vi "Day 13.vi"() -> ()   [LabVIEW 2021]
panel:
  out "output 2":bool[][](array[boolean])
  out "input":string
  out "input file":path
  in  "Run [T]/ Example[F]":bool
  out "ouptut 1":u32
  # "Advent of Code 2021 - Day 11 - Dumbo Octopus"
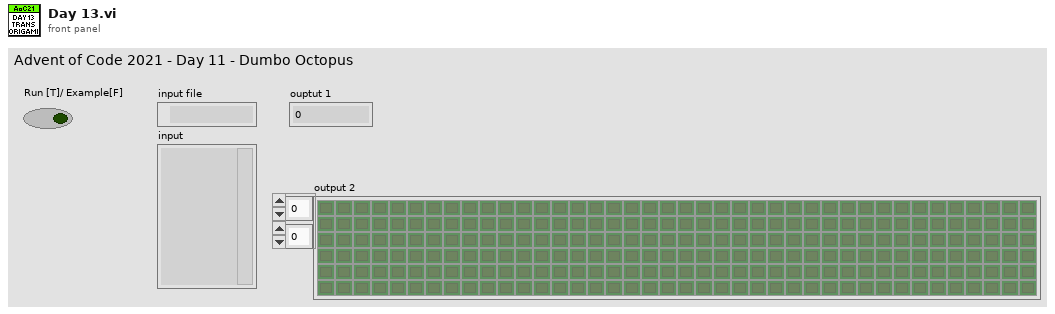
[diagram p1: front panel]
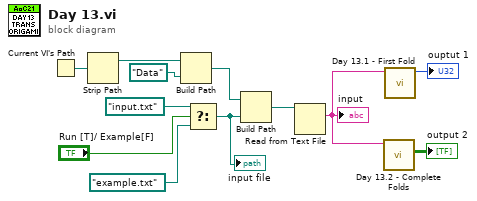
[diagram p0: block diagram]
diagram:
  n1 = Current VI's Path() -> (path=w12:path)
  n2 = Strip Path(path=w12) -> (stripped path=w11:path)  [unwired: 1 out]
  n3 = Build Path(base path=w11, name or relative path=path "Data") -> (appended path=w9:path)
  n4 = Select(t=path "input.txt" ("name or relative path"), s="Run [T]/ Example[F]", f=path "example.txt" ("name or relative path")) -> (s? t:f=w5:path)
  "input file" <- w5
  n5 = Build Path(base path=w9, name or relative path=w5) -> (appended path=w3:path)
  n6 = Read from Text File(file (use dialog)=w3) -> (text=w2:string)  [unwired: 3 in, 3 out]
  "input" <- w2
  n7 = call "Day 13.2 - Complete Folds.vi"("input"=w2) -> ("output array"=→"output 2":bool[][])  [unwired: 9 in, 1 out]
  n8 = call "Day 13.1 - First Fold.vi"("input"=w2) -> ("output"=→"ouptut 1":i32)  [unwired: 10 in]
